vi "Point Array to Polygon Points.vi"(8 "error in (no error)":errorcluster, 11 "Point Array":T1[](array[typedef])=[{"Longitude"=0.0, "Latitude"=0.0}] {"Latitude" format="%#_10g"; "Longitude" format="%#_10g"}) -> (0 "error out":errorcluster, 3 "Polygon Points":refnum<k24>)   [LabVIEW 2014]
uses:
  Lat Long Conversion/Controls/PointLatLon.ctl
  C:/Robotic Systems/Products/AgFalcon/Software/Ground Station/Data/Mapping DLL/GMap.NET.Core.dll
  Data/Mapping DLL/GMap.NET.Core.dll
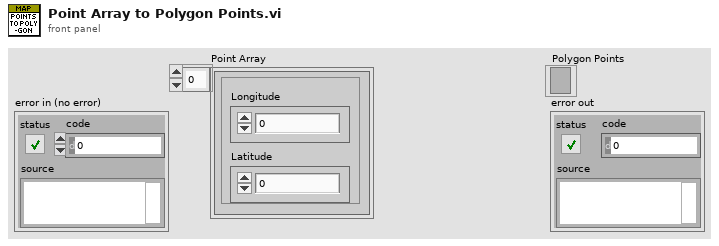
[diagram p1: front panel]
types:
  T1 = typedef "PointLatLon.ctl" = cluster{"Longitude":dbl, "Latitude":dbl}
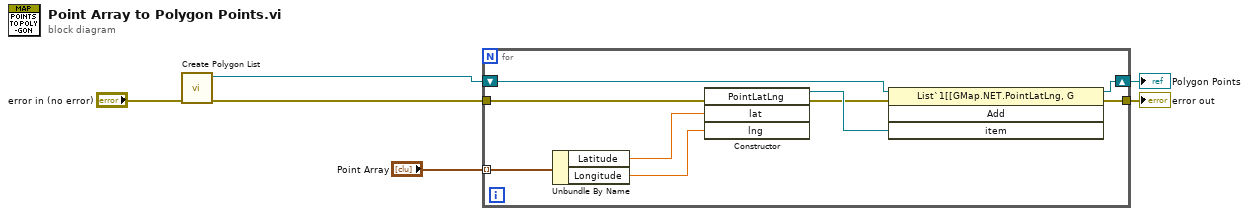
[diagram p0: block diagram]
diagram:
  n1 = call "Create Polygon List.vi"("error in (no error)"="error in (no error)") -> ("error out"=w5:errorcluster, "specific class reference"=w6:refnum<k24>)  [unwired: 9 in]
  n2 = for {
    tunnel: w5 -> [w9]
    shift-right: [w14] -> w4
    shift-left: w6 -> [w15]
    tunnel: [w13] -> w3
    tunnel: "Point Array" -> [w12] mode=indexing
    n3 = Unbundle By Name(w12) -> ("Latitude"=w11:dbl, "Longitude"=w10:dbl)
    n4 = constructor class="PointLatLng"(error in=w9, "lat"=w11, "lng"=w10) -> (reference out=w8:refnum<k24>, error out=w7:errorcluster)  [unwired: 2 in, 3 out]
    n5 = invoke class="List`1[[GMap.NET.PointLatLng, G" method="Add"(reference=w15, error in=w7, "item"=w8) -> (reference out=w14:refnum<k24>, error out=w13:errorcluster)  [unwired: 1 in, 2 out]
  }
  "Polygon Points" <- w4
  "error out" <- w3
